vi "Read Spec Page Path.vi"(8 "error in (no error)":errorcluster, 11 "MetaDataObj in":refnum<class "MetaDataObj.lvclass">) -> (0 "error out":errorcluster, 2 "Path to Spec Page VI":path, 3 "MetaDataObj out":refnum<class "MetaDataObj.lvclass">)   [LabVIEW 2016, in "MetaDataObj.lvclass"]
uses:
  <resource>/dialog/NewProjectWizard/MetaDataObj/MetaDataObj.lvclass
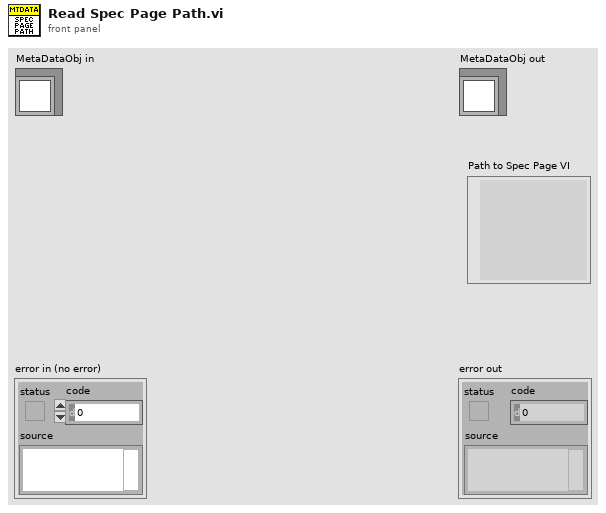
[diagram p1: front panel]
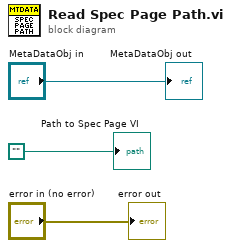
[diagram p0: block diagram]
diagram:
  "error out" <- "error in (no error)"
  "MetaDataObj out" <- "MetaDataObj in"
  "Path to Spec Page VI" <- path ""
